vi "Try Parse.vi"(0 "Vector Path in":refnum<class "Vector 18GHz Path.lvclass">, 5 "Config Row":string[](array[string]), 11 "error in":errorcluster) -> (4 "Vector Path out":refnum<class "Vector 18GHz Path.lvclass">, 6 "Is of type?":bool, 15 "error out":errorcluster)   [LabVIEW 2023, in "RFFixtureCharact.RFPM.lvlib" / "Vector 18GHz Path.lvclass"]
uses:
  Vector 18GHz Path.lvclass
  Vector 18GHz Path.lvclass/Vector 18GHz Path.ctl
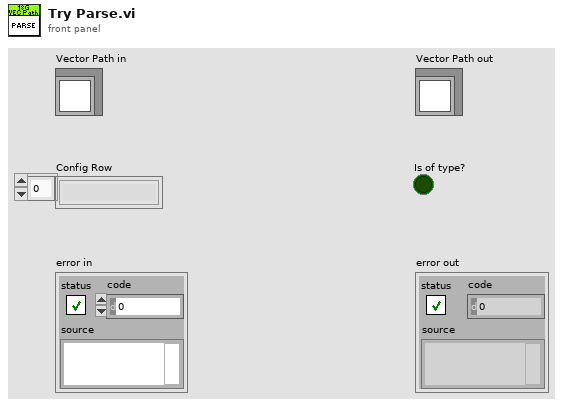
[diagram p1: front panel]
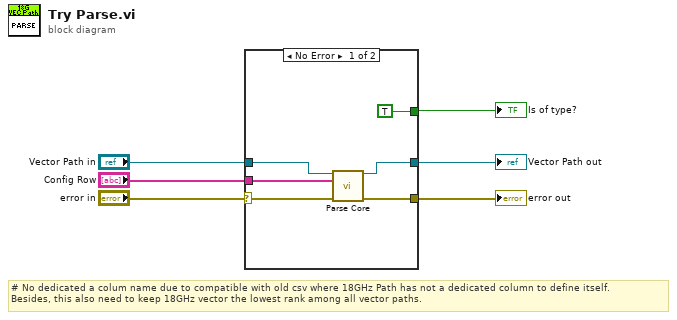
[diagram p0: block diagram]
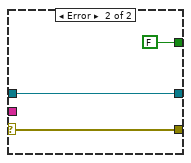
[diagram p2: hidden frame]
diagram:
  # "# No dedicated a colum name due to compatible with old csv where 18GHz Path has not a dedicated column to define itself.\nBesides, this also need to keep 18GHz vector the lowest rank among all vector paths."
  n1 = case shown="No Error" "error in" {
    selector: "error in" -> [w7 w15]
    tunnel: [w8 w15] -> w1
    tunnel: [TRUE ("Is of type?") FALSE ("Is of type?")] -> w3
    tunnel: [w9 w14] -> w2
    tunnel: "Config Row" -> [w10 _]
    tunnel: "Vector Path in" -> [w11 w14]
    frame No Error {
      n2 = call-dynamic "Parse Core.vi"("Vector Path in"=w11, "Config Row"=w10, "error in"=w7) -> ("Vector Path out"=w9:refnum<class "Vector 18GHz Path.lvclass">, "error out"=w8:errorcluster)  [unwired: 11 in]
    }
    frame Error {
    }
  }
  "error out" <- w1
  "Vector Path out" <- w2
  "Is of type?" <- w3
